vi "3.vi"() -> ()   [LabVIEW 2018]
uses:
  D:/LABVIEW/examples/Instrument IO/Serial/support/Serial - Settings.ctl
  D:/LABVIEW/examples/Instrument IO/Serial/support/Serial - XON-XOFF Characters.ctl
  D:/LABVIEW/examples/Instrument IO/Serial/support/Serial - ASCII Characters.ctl
  <vilib>/Instr/_visa.llb/VISA Configure Serial Port (Instr).vi
panel:
  out "接收到的":string
  out "判断":string
  in  "XON/XOFF校验字符":T1={"XON"=enum."DC1", "XOFF"=enum."DC3"}
  in  "串口设置":T3={"波特率"=9600, "数据位"=8, "校验"=enum."None", "停止位"=10, "流控制"=0} {"流控制" items=["无"=0, "XON/XOFF"=1, "RTS/CTS"=2, "DTR/DSR"=4]; "停止位" items=["1.0"=10, "1.5"=15, "2.0"=20]; "数据位" min=5 max=8 step=1; "波特率" items=["75"=75, "110"=110, "134"=134, "150"=150, "300"=300, "600"=600, "1200"=1200, "1800"=1800, "2400"=2400, "4800"=4800, "7200"=7200, "9600"=9600, "14400"=14400, "19200"=19200, "28800"=28800, "38400"=38400, "56000"=56000, "57600"=57600, "115200"=115200, "128000"=128000, "230400"=230400]}
  in  "串口资源":refnum<visa-resource-name>="COM1"
  in  "停止":bool
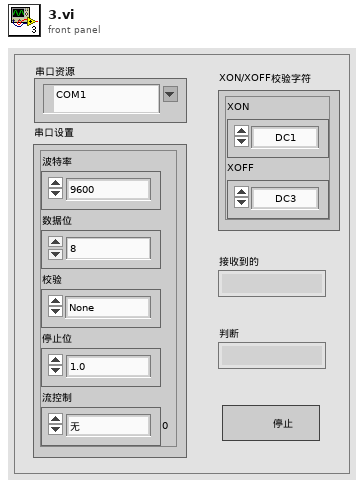
[diagram p1: front panel]
types:
  T1 = typedef "Serial - XON-XOFF Characters.ctl" = cluster{"XON":T2, "XOFF":T2}
  T2 = typedef "Serial - ASCII Characters.ctl" = enum16{"NUL", "SOH", "STX", "ETX", "EOT", "ENQ", "ACK", "BEL", "BS", "HT", "LF", "VT", "FF", "CR", "SO", "SI", "DLE", "DC1", "DC2", "DC3", "DC4", "NAK", "SYN", "ETB", "CAN", "EM", "SUB", "ESC", "FS", "GS", "RS", "US", "SP", "!", "\"", "#", "$", "%", "&", "'", "(", ")", "*", "+", ",", "- (-)", ".", "/", "0", "1", "2", "3", "4", "5", "6", "7", "8", "9", ":", ";", "<", "=", ">", "?", "@", "A", "B", "C", "D", "E", "F", "G", "H", "I", "J", "K", "L", "M", "N", "O", "P", "Q", "R", "S", "T", "U", "V", "W", "X", "Y", "Z", "[", "\\", "]", "^", "_", "`", "a", "b", "c", "d", "e", "f", "g", "h", "i", "j", "k", "l", "m", "n", "o", "p", "q", "r", "s", "t", "u", "v", "w", "x", "y", "z", "{", "|", "}", "~"}
  T3 = typedef "Serial - Settings.ctl" = cluster{"波特率":u32, "数据位":u16, "校验":enum16{"None", "Odd", "Even", "Mark", "Space"}, "停止位":u16, "流控制":u16}
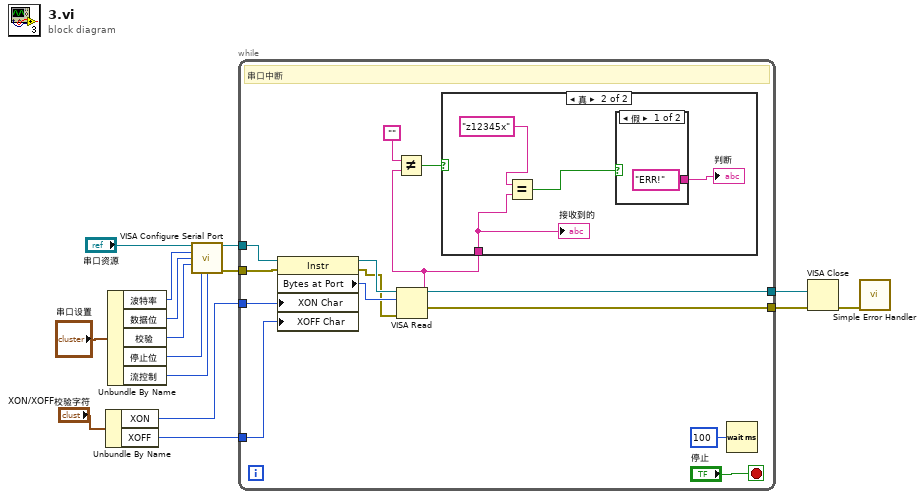
[diagram p0: block diagram]
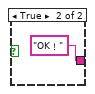
[diagram p3: hidden frame]
diagram:
  n1 = Unbundle By Name("XON/XOFF校验字符") -> ("XON"=w5:T2, "XOFF"=w4:T2)
  n2 = Unbundle By Name("串口设置") -> ("波特率"=w13:u32, "数据位"=w12:u16, "校验"=w11:enum16{"None", "Odd", "Even", "Mark", "Space"}, "停止位"=w10:u16, "流控制"=w9:u16)
  n3 = call-poly "VISA Configure Serial Port"("VISA resource name"="串口资源", "baud rate (9600)"=w13, "data bits (8)"=w12, "parity (0:none)"=w11, "stop bits (10: 1 bit)"=w10, "flow control (0:none)"=w9) -> ("VISA resource name out"=w7:refnum<visa-resource-name>, "error out"=w8:errorcluster)  [unwired: 3 in, 5 out]
  n4 = while {
    tunnel: w7 -> [w29]
    tunnel: w8 -> [w28]
    tunnel: w5 -> [w25]
    tunnel: w4 -> [w24]
    tunnel: [w20] -> w2
    tunnel: [w19] -> w1
    stop <- "停止" stop-if-true
    # "串口中断"
    n5 = property class="Instr"(reference=w29, error in=w28, "XON Char"=w25, "XOFF Char"=w24) -> (reference out=w22:refnum<visa-resource-name>, error out=w21:errorcluster, "Bytes at Port"=w23:u32)
    n6 = VISA Read(VISA resource name=w22, byte count=w23, error in (no error)=w21) -> (VISA resource name out=w20:refnum<visa-resource-name>, read buffer=w17:string, error out=w19:errorcluster)  [unwired: 1 out]
    n7 = Not Equal?(x="", y=w17) -> (x != y?=w16:bool)
    n8 = case shown="真" w16 {
      tunnel: w17 -> [_ w30]
      frame False {
      }
      frame True {
        n9 = Equal?(x="z12345x", y=w30) -> (x = y?=w32:bool)
        n10 = case shown="假" w32 {
          tunnel: ["ERR!" "OK！"] -> w31
          frame False {
          }
          frame True {
          }
        }
        "判断" <- w31
        "接收到的" <- w30
      }
    }
    n11 = Wait (ms)(milliseconds to wait=u32 100) -> ()  [unwired: 1 out]
  }
  n12 = VISA Close(VISA resource name=w2, error in (no error)=w1) -> (error out=w3:errorcluster)
  n13 = call <vilib>:"Simple Error Handler.vi"("error in (no error)"=w3) -> ()  [unwired: 1 in, 8 out]
